vi "Preview_Build.vi"(8 "error in (no error)":errorcluster, 11 "Build in":refnum<class "AB_InteropAssembly.lvclass">) -> (0 "error out":errorcluster, 1 "GeneratedFiles":path[](array[path]), 3 "Build out":refnum<class "AB_InteropAssembly.lvclass">, 4 "GeneratedFileGUIDs":string[](array[string]), 5 "OutputDirectory":path)   [LabVIEW 2020, in "AB_InteropAssembly.lvclass"]
uses:
  <vilib>/AppBuilder/AB_Classes/InteropAssembly/AB_InteropAssembly.lvclass
  e:/builds/penguin/labview/branches/2020/dev/dist/vi.lib/AppBuilder/AB_Classes/Build/AB_Build.lvclass
  <vilib>/AppBuilder/AB_Classes/Application/AB_Application.lvclass
  <vilib>/AppBuilder/AB_Classes/Build/AB_Build.lvclass
  <vilib>/AppBuilder/AB_Classes/Destination/AB_Destination.lvclass
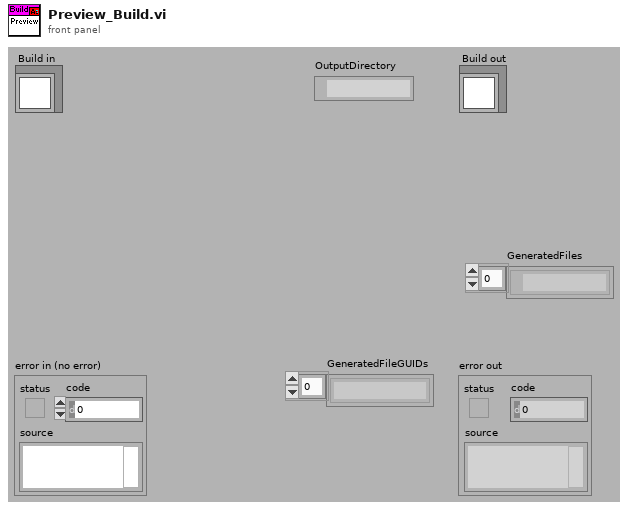
[diagram p1: front panel]
types:
  T1 = typedef "AB_Build.ctl" = cluster{"buildSpecName":string, "buildSpecDescription":string, "destinations":refnum<class "AB_Destination.lvclass">[], "exclusionOption":T2, "defaultLanguage":string, "supportedLanguages":string[], "excludedDirectories":path[], "buildContext":refnum<vi>, "buildObject":T3, "preview":bool, "programatic":bool, "progressBarEvents":T4, "userLog_Path":path, "preActionID":string, "preAction_Path":path, "postActionID":string, "postAction_Path":path, "eng_checkForBrokenVIs?":bool, "eng_verboseLinkerErrors?":bool, "localDest_Path":path, "targetDest_Path":path, "removeVIObject":u16, "cache":refnum<class "PreviewCache.lvclass">, "use cache":bool, "previewCache_ID":string, "buildCache_ID":string, "eng_TempLocalDest_Path":path, "eng_collectDependencies?":bool, "versionInfo":cluster{"buildVersion":cluster{"major":u16, "minor":u16, "patch":u16, "build":u16}, "autoIncrement":bool}, "eng_enableVIChecksums":bool}
  T2 = typedef "AB_Exclusion_Option.ctl" = cluster{"typedefs":bool, "polymorphicVIs":bool, "unusedLibraryItems":bool, "modifyLibraryFile":bool, "edit-timeDependencies":bool, "inlineVIs":bool, "dependent PPLs":bool, "dependent DLLs":bool}
  T3 = typedef "ItemRef.ctl" = u64
  T4 = typedef "provcom_ProgressBar_Events.ctl" = cluster{"newJob":refnum<user-event>, "newItem":refnum<user-event>, "errorMsg":T5, "cancel":refnum<user-event>}
  T5 = typedef "mxLvBuildError.ctl" = refnum<user-event>
  T6 = typedef "AB_Destination.ctl" = cluster{"destName":string, "path":path, "libraryName":string, "preserveHierarchy":bool, "eng_inBuild":bool, "eng_libraryReference":refnum<vi>, "eng_restictAddToNewLibrary":bool}
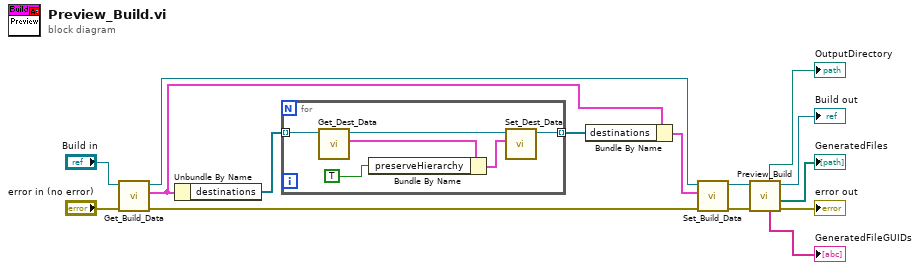
[diagram p0: block diagram]
diagram:
  n1 = call <vilib>:"Get_Build_Data.vi"("error in (no error)"="error in (no error)", "Class in"="Build in") -> ("error out"=w2:errorcluster, "data"=w8:T1, "Class out"=w6:refnum<class "AB_InteropAssembly.lvclass">)  [unwired: 7 out]
  n2 = Unbundle By Name(w8) -> ("destinations"=w9:refnum<class "AB_Destination.lvclass">[])
  n3 = for {
    tunnel: w9 -> [w16] mode=indexing
    tunnel: [w17] -> w4 mode=indexing
    n4 = call <vilib>:"Get_Dest_Data.vi"("Class in"=w16) -> ("destName"=w21:T6, "Class out"=w18:refnum<class "AB_Destination.lvclass">)  [unwired: 8 in, 1 out]
    n5 = Bundle By Name(cluster=w21, "preserveHierarchy"=TRUE) -> (w19:T6)
    n6 = call <vilib>:"Set_Dest_Data.vi"("destName"=w19, "Class in"=w18) -> ("Class out"=w17:refnum<class "AB_Destination.lvclass">)  [unwired: 8 in, 1 out]
  }
  n7 = Bundle By Name(cluster=w8, "destinations"=w4) -> (w7:T1)
  n8 = call <vilib>:"Set_Build_Data.vi"("error in (no error)"=w2, "data"=w7, "Class in"=w6) -> ("error out"=w1:errorcluster, "Class out"=w5:refnum<class "AB_InteropAssembly.lvclass">)  [unwired: 7 in]
  n9 = call-parent "Preview_Build.vi"("error in (no error)"=w1, "Build in"=w5) -> ("error out"=→"error out":errorcluster, "GeneratedFiles"=→"GeneratedFiles":path[], "Build out"=→"Build out":refnum<class "AB_InteropAssembly.lvclass">, "GeneratedFileGUIDs"=→"GeneratedFileGUIDs":string[], "OutputDirectory"=→"OutputDirectory":path)  [unwired: 5 in]
